vi "HovaCAL reset after purge.vi"(8 "Fehler (Eingang, kein Fehler)":errorcluster) -> (0 "Fehler (Ausgang)":errorcluster)   [LabVIEW 2020, in "EPA 1065.lvlib" / "HovaCAL Interference verificaton.lvlib"]
uses:
  Linearisierung V2/Gasteiler/HovaCAL_Interface/Kommunikation/Aktion_FGV_HovaCAL_Interface_Kommandos.ctl
  Linearisierung V2/Gasteiler/HovaCAL_Interface/Kommunikation/Aktion_FGV_HovaCAL_Interface_Kommunikation.ctl
  Aktion FGV Interference.ctl
  HovaCAL Interference verificaton.lvlib
  Linearisierung V2/Gasteiler/HovaCAL_Interface/Kommunikation/Kommunikation.lvlib
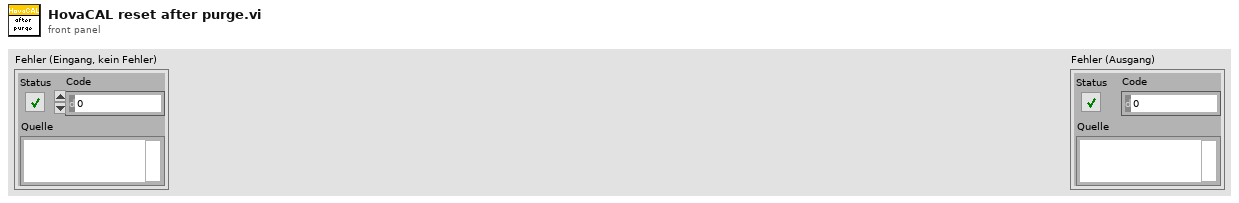
[diagram p1: front panel]
types:
  T1 = typedef "EPA 1065.lvlib/HovaCAL Interference verificaton.lvlib/Aktion FGV Interference.ctl" = enum16{"Lesen", "TestKonfig", "TestSetting", "Einheiten", "Ergebnis", "Laden", "Tabelle", "Speichern", "löschen"}
  T2 = typedef "Linearisierung v2.lvlib/Gasteiler.lvlib/HovaCAL_Interface.lvlib/Kommunikation.lvlib/Aktion_FGV_HovaCAL_Interface_Kommunikation.ctl" = enum16{"Initialisieren", "Set Konzentrationen", "Set Gase", "Set Limits", "Get Dynamische Werte", "Beenden", "Com ändern", "Get Gase init", "Pause", "Get Gasteiler Infos", "Get MFC Infos", "Set Pumpen Parameter", "Set Pumpe Konzenration", "Set Pumpe run", "Set Temperaturen", "Set Fluss", "Get Gase", "Get Limits", "Get Dynamische Werte 1", "Get Dynamische Werte 2"}
  T3 = typedef "Linearisierung v2.lvlib/Gasteiler.lvlib/HovaCAL_Interface.lvlib/Kommunikation.lvlib/Aktion_FGV_HovaCAL_Interface_Kommandos.ctl" = enum16{"lesen", "verarbeiten", "hinzufügen", "on top", "init", "sammeln", "freigeben", "connected"}
  T4 = typedef "EPA 1065.lvlib/HovaCAL Interference verificaton.lvlib/TestKonfig.ctl" = cluster{"TestKonfig H2O":T5, "TestKonfig Interferent":T11}
  T5 = typedef "EPA 1065.lvlib/HovaCAL Interference verificaton.lvlib/TestKonfig H2O.ctl" = cluster{"Modus":T6, "Komponente:":u16, "Eingangs Konzentration:":dbl, "Einheit":T7, "Anzahl Stufen":sgl, "Zeitdauer Stufen":sgl, "Max Fehler":sgl, "zusätzliche Zeitdauer Erster Punkt":sgl, "Punkte umkehren":bool, "Stufen Tabelle":T8, "HovaCAL Flow Input Cluster":T9, "HovaCAL Temperature":T10}
  T6 = typedef "EPA 1065.lvlib/HovaCAL Interference verificaton.lvlib/Modus.ctl" = u16
  T7 = typedef "Linearisierung v2.lvlib/SpanEinstellungen.lvlib/Einheit.ctl" = enum16{"ppm", "%"}
  T8 = typedef "Linearisierung v2.lvlib/Gasteiler.lvlib/Stufen Tabelle 10 Stufen.ctl" = string[][]
  T9 = typedef "Linearisierung v2.lvlib/Gasteiler.lvlib/HovaCAL_Interface.lvlib/Controls.lvlib/Flow Einstellung.ctl" = cluster{"HovaCAL Flow Input Cluster":dbl}
  T10 = typedef "Linearisierung v2.lvlib/Gasteiler.lvlib/HovaCAL_Interface.lvlib/Controls.lvlib/Temp Sollwerte Anzeige.ctl" = dbl[]
  T11 = typedef "EPA 1065.lvlib/HovaCAL Interference verificaton.lvlib/TestKonfig Interferents.ctl" = cluster{"MFC1":enum16{"MFC 1"}, "Eingangs Konzentration MFC1":dbl, "Einheit MFC1 Eingang":T7, "Ausgangs Konzentration MFC1":dbl, "Einheit MFC1 Ausgang":T7, "MFC2":T12, "Referenz-Interferent:":u16, "Gasflaschen Nr MFC2":string, "Accuracy MFC2":string, "Eingangs Konzentration MFC2":dbl, "Einheit MFC2 Eingang":T7, "Ausgangs Konzentration MFC2":dbl, "Einheit MFC2 Ausgang":T7, "MFC3":T12, "Kontroll-Interferent:":u16, "Gasflaschen Nr MFC3":string, "Accuracy MFC3":string, "Eingangs Konzentration MFC3":dbl, "Einheit MFC3 Eingang":T7, "Ausgangs Konzentration MFC3":dbl, "Einheit MFC3 Ausgang":T7, "Gasflasche MFC2":T13, "Gasflasche MFC3":T13}
  T12 = typedef "EPA 1065.lvlib/HovaCAL Interference verificaton.lvlib/MFCAuswahl.ctl" = u16
  T13 = typedef "System Einstellungen V2.lvlib/Gasflasche Auswahl.ctl" = u16
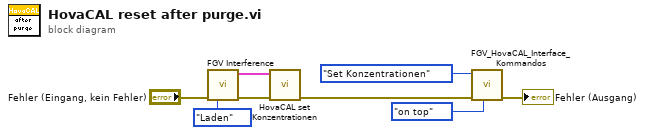
[diagram p0: block diagram]
diagram:
  n1 = call "FGV Interference.vi"("error in (no error)"="Fehler (Eingang, kein Fehler)", "Aktion FGV Interference"=Aktion_FGV_Interference."Laden") -> ("TestKonfig"=w2:T4, "error out"=w4:errorcluster)  [unwired: 8 in, 4 out]
  n2 = call "HovaCAL set Konzentrationen.vi"("Fehler (Eingang, kein Fehler)"=w4, "TestKonfig (Eingang)"=w2) -> ("Fehler (Ausgang)"=w3:errorcluster)  [unwired: 9 in]
  n3 = call "FGV_HovaCAL_Interface_Kommandos.vi"("Aktion"=Aktion_FGV_HovaCAL_Interface_Kommandos."on top", "error in"=w3, "Kommando in"=Aktion_FGV_HovaCAL_Interface_Kommunikation."Set Konzentrationen") -> ("error out"=→"Fehler (Ausgang)":errorcluster)  [unwired: 2 in, 5 out]
